vi "svl_Maximum Sound Level (N Ch).vi"(6 "restart averaging (F)":bool, 8 "error in (no error)":errorcluster, 11 "scaled signals":waveform(dbl)[](array[waveform])) -> (0 "error out":errorcluster, 3 "maximum sound levels [dB EU]":dbl[](array[numeric]) format="%.2f")   [LabVIEW 2017]
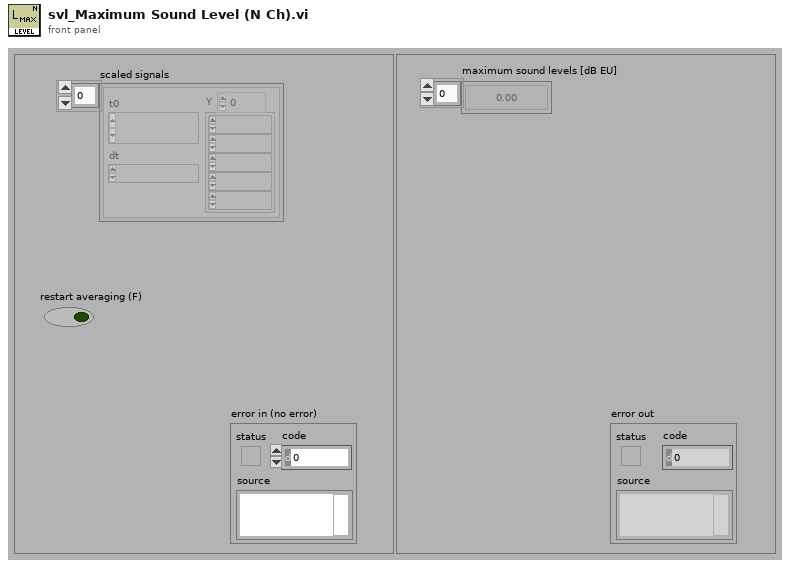
[diagram p1: front panel]
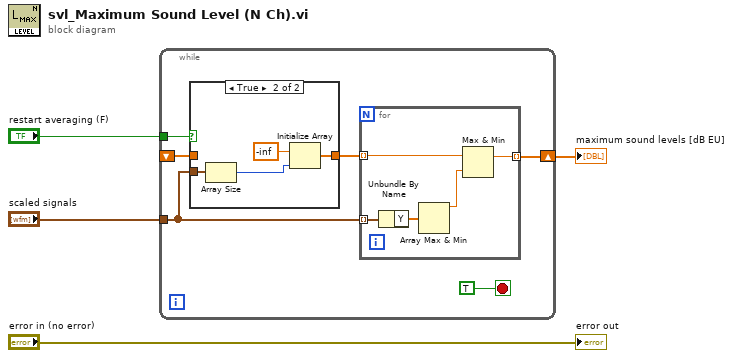
[diagram p0: block diagram]
diagram:
  n1 = while {
    shift-right: [w5] -> w1
    shift-left: _ -> [w7]
    tunnel: "restart averaging (F)" -> [w9]
    tunnel: "scaled signals" -> [w6]
    stop <- TRUE stop-if-true
    n2 = case shown="True" w9 {
      tunnel: w6 -> [_ w15]
      tunnel: [w11 w13] -> w8
      tunnel: w7 -> [w11 _]
      frame False {
      }
      frame True {
        n3 = Array Size(array=w15) -> (size(s)=w12:i32)
        n4 = Initialize Array(-inf ("element"), w12) -> (w13:dbl[])
      }
    }
    n5 = for {
      tunnel: w8 -> [w19] mode=indexing
      tunnel: w6 -> [w17] mode=indexing
      tunnel: [w18] -> w5 mode=indexing
      n6 = Unbundle By Name(w17) -> ("Y"=w16:dbl[])
      n7 = Array Max & Min(array=w16) -> (max value=w20:dbl)  [unwired: 3 out]
      n8 = Max & Min(x=w19, y=w20) -> (max(x,y)=w18:dbl)  [unwired: 1 out]
    }
  }
  "maximum sound levels [dB EU]" <- w1
  "error out" <- "error in (no error)"
